vi "Item BG Color.vi"(0 "Tree Reference In":refnum<vi>, 1 "Tag (Current)":string, 2 "Cell BG Color":u32(colorbox)=16777226, 5 "error in (no error)":errorcluster) -> (14 "Tree Reference Out":refnum<vi>, 15 "Duplicate Tag":string, 19 "error out":errorcluster)   [LabVIEW 2012, in "QuickVIew.lvlib"]
doc: "Sets cell BG color"
uses:
  QuickVIew.lvlib
panel:
  # "VI INPUTS"
  # "VI OUTPUTS"
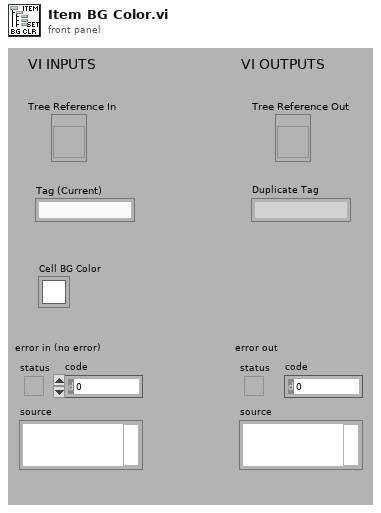
[diagram p1: front panel]
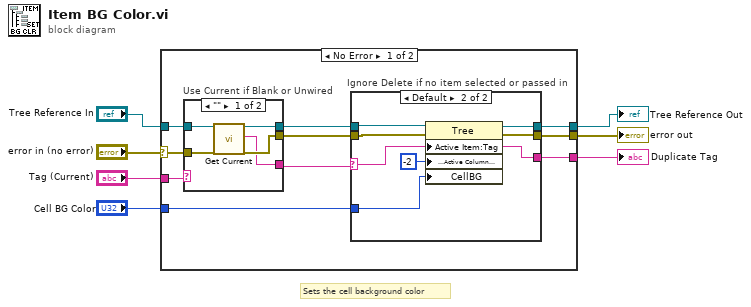
[diagram p0: block diagram]
diagram:
  # "Sets the cell background color"
  n1 = case shown="No Error" "error in (no error)" {
    selector: "error in (no error)" -> [w15 w37]
    tunnel: "Tree Reference In" -> [w17 w38]
    tunnel: [w14 w38] -> w6
    tunnel: [w13 w37] -> w5
    tunnel: "Tag (Current)" -> [w16 w36]
    tunnel: "Cell BG Color" -> [w9 _]
    tunnel: [w8 w36] -> w1
    frame No Error {
      n2 = case "Use Current if Blank or Unwired" shown="\"\"" w16 {
        selector: w16 -> [_ w33]
        tunnel: [w31 w35] -> w12
        tunnel: w17 -> [w32 w35]
        tunnel: [w30 w34] -> w11
        tunnel: w15 -> [w29 w34]
        tunnel: [w28 w33] -> w10
        frame "" {
          n3 = call "Get Current.vi"("Tree Reference In"=w32, "error in (no error)"=w29) -> ("Tree Reference Out"=w31:refnum<vi>, "Current Tag"=w28:string, "error out"=w30:errorcluster)  [unwired: 14 in, 1 out]
        }
        frame Default {
        }
      }
      n4 = case "Ignore Delete if no item selected or passed in" shown="Default" w10 {
        selector: w10 -> [w18 w23]
        tunnel: [w20 w25] -> w14
        tunnel: [w19 w24] -> w13
        tunnel: w12 -> [w20 w27]
        tunnel: w11 -> [w19 w26]
        tunnel: w9 -> [_ w21]
        tunnel: [w18 w23] -> w8
        frame "" {
        }
        frame Default {
          n5 = property class="Tree"(reference=w27, error in=w26, "Active Item:Tag"=w23, "Active Cell:Active Column Number"=-2, "CellBG"=w21) -> (reference out=w25:refnum<vi>, error out=w24:errorcluster)
        }
      }
    }
    frame Error {
    }
  }
  "Tree Reference Out" <- w6
  "error out" <- w5
  "Duplicate Tag" <- w1
